vi "BeadCooler(SubVI).vi"(0 "Enum":T1(ring), 1 "Input":i16, 2 "Setpoint":fxp<+/-,16,16>, 3 "drive":fxp<+/-,32,16>, 7 "dg":fxp<+/-,32,16>, 9 "pg":fxp<+/-,32,16>, 12 "Dc offset":fxp<+/-,32,16>, 13 "Upper lim":fxp<+/-,32,16>, 14 "Lower lim":fxp<+/-,32,16>) -> (6 "Output":fxp<+/-,32,16>)   [LabVIEW 2013]
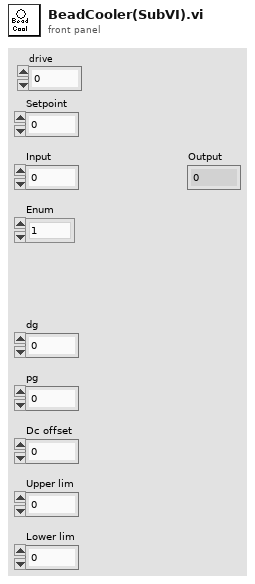
[diagram p1: front panel]
types:
  T1 = enum16{"1", "2", "4", "8", "16", "32", "64", "128", "256", "512"}
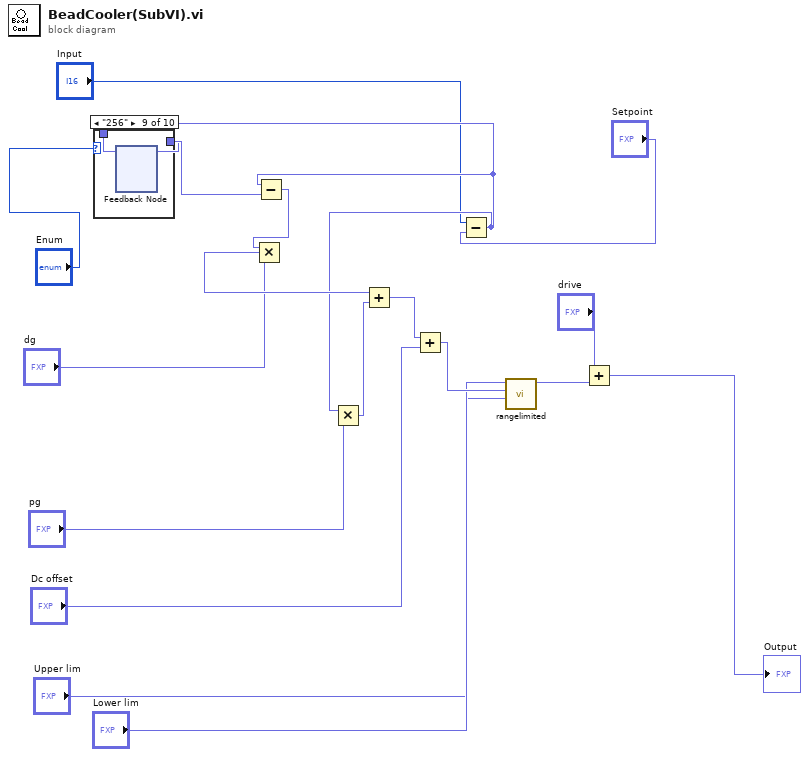
[diagram p0: block diagram]
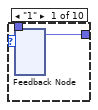
[diagram p2: hidden frame]
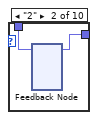
[diagram p3: hidden frame]
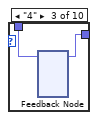
[diagram p4: hidden frame]
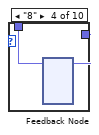
[diagram p5: hidden frame]
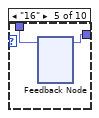
[diagram p6: hidden frame]
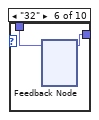
[diagram p7: hidden frame]
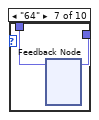
[diagram p8: hidden frame]
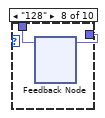
[diagram p9: hidden frame]
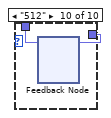
[diagram p10: hidden frame]
diagram:
  n1 = Subtract(x="Input", y="Setpoint") -> (x-y=w7:fxp<+/-,17,17>)
  n2 = case shown="\"256\"" "Enum" {
    tunnel: [w20 w21 w23 w25 w27 w29 w31 w33 w35 w37] -> w11
    tunnel: w7 -> [w19 w22 w24 w26 w28 w30 w32 w34 w36 w38]
    frame "1" {
      n3 = feedback #1() -> (w20:fxp<+/-,17,17>)  [unwired: 1 in]
      n4 = feedback-in #1(w19) -> ()
    }
    frame "2" {
      n5 = feedback #2() -> (w21:fxp<+/-,17,17>)  [unwired: 1 in]
      n6 = feedback-in #2(w22) -> ()
    }
    frame "4" {
      n7 = feedback #3() -> (w23:fxp<+/-,17,17>)  [unwired: 1 in]
      n8 = feedback-in #3(w24) -> ()
    }
    frame "8" {
      n9 = feedback #4() -> (w25:fxp<+/-,17,17>)  [unwired: 1 in]
      n10 = feedback-in #4(w26) -> ()
    }
    frame "16" {
      n11 = feedback #5() -> (w27:fxp<+/-,17,17>)  [unwired: 1 in]
      n12 = feedback-in #5(w28) -> ()
    }
    frame "32" {
      n13 = feedback #6() -> (w29:fxp<+/-,17,17>)  [unwired: 1 in]
      n14 = feedback-in #6(w30) -> ()
    }
    frame "64" {
      n15 = feedback #7() -> (w31:fxp<+/-,17,17>)  [unwired: 1 in]
      n16 = feedback-in #7(w32) -> ()
    }
    frame "128" {
      n17 = feedback #8() -> (w33:fxp<+/-,17,17>)  [unwired: 1 in]
      n18 = feedback-in #8(w34) -> ()
    }
    frame "256" {
      n19 = feedback #9() -> (w35:fxp<+/-,17,17>)  [unwired: 1 in]
      n20 = feedback-in #9(w36) -> ()
    }
    frame "512" {
      n21 = feedback #10() -> (w37:fxp<+/-,17,17>)  [unwired: 1 in]
      n22 = feedback-in #10(w38) -> ()
    }
  }
  n23 = Subtract(x=w7, y=w11) -> (x-y=w12:fxp<+/-,18,18>)
  n24 = Multiply(x=w12, y="dg") -> (x*y=w18:fxp<+/-,49,33>)
  n25 = Multiply(x=w7, y="pg") -> (x*y=w15:fxp<+/-,48,32>)
  n26 = Add(x=w18, y=w15) -> (x+y=w4:fxp<+/-,50,34>)
  n27 = Add(x=w4, y="Dc offset") -> (x+y=w17:fxp<+/-,50,34>)
  n28 = call "rangelimited.vi"("Upper lim"="Upper lim", "Input"=w17, "Lower lim"="Lower lim") -> ("Output"=w3:fxp<+/-,32,16>)  [unwired: 8 in]
  n29 = Add(x="drive", y=w3) -> (x+y=→"Output":fxp<+/-,33,17>)
